vi "Auswerten.vi"(7 "Êinheiten":string[](array[string]), 8 "LIN Ausgabetabelle":refnum<vi>, 9 "Komponente:":refnum<vi>, 10 "max. Flow Weighted Mean:":refnum<vi>, 11 "Tabelle":T1[][](array[typedef])) -> (0 "Konzentration Komponente":dbl, 1 "Komponente:":T1, 2 "max. Flow Weighted Mean:":T1, 3 "Konzentration FlowWeightedMean":dbl)   [LabVIEW 2020, in "EPA 1065.lvlib" / "Interference verificaton 1065-375.lvlib"]
uses:
  Interference verificaton 1065-375.lvlib
  Visualisierungs Elemente/String - Ausgabefeld.ctl
  <vilib>/Utility/miscctls.llb/LVRowAndColumnTypeDef.ctl
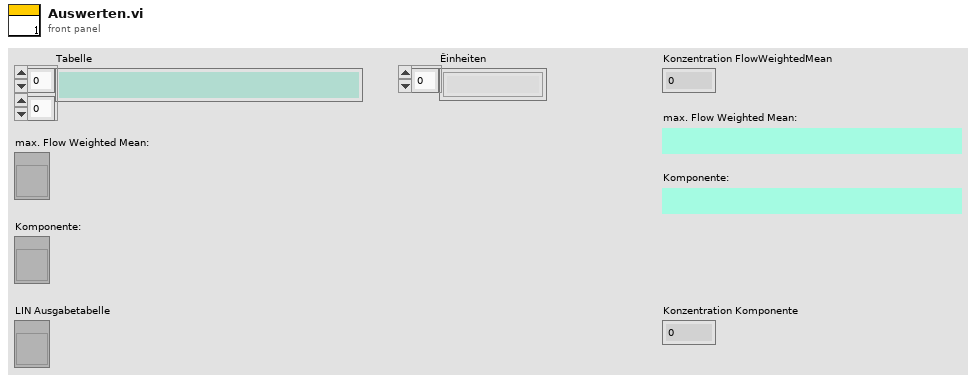
[diagram p1: front panel]
types:
  T1 = typedef "String - Ausgabefeld.ctl" = string
  T2 = typedef "LVRowAndColumnTypeDef.ctl" = cluster{"Row":i32, "Column":i32}
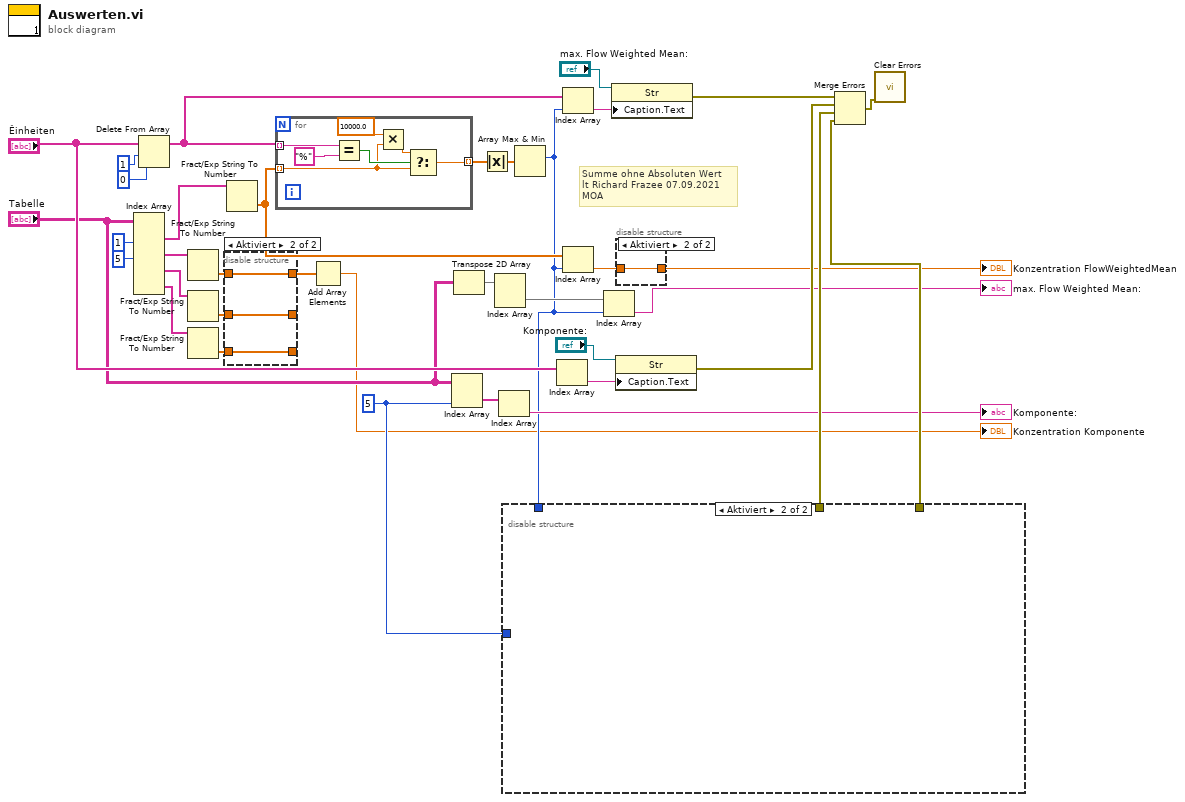
[diagram p0: block diagram]
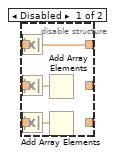
[diagram p2: hidden frame]
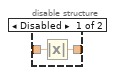
[diagram p3: hidden frame]
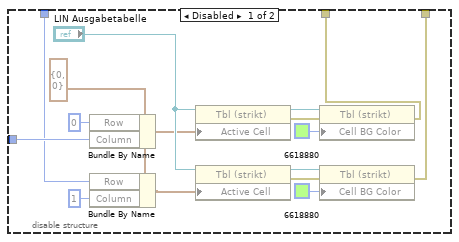
[diagram p4: hidden frame]
diagram:
  w32 = 5 ("y")
  # "Summe ohne Absoluten Wert \nlt Richard Frazee 07.09.2021\nMOA"
  n1 = Index Array(array="Tabelle", index (col) #1=1 ("Deaktivierter Index (Spalte)"), index (col) #2=5 ("Index (Spalte)")) -> (element #1=w10:T1[], element #2=w11:T1[], element #3=w14:T1[], element #4=w16:T1[])  [unwired: 6 in]
  n2 = Delete From Array(array="Êinheiten", length=1 ("Länge"), index=0 ("Index")) -> (array with subset deleted=w18:string[])  [unwired: 1 out]
  n3 = Fract/Exp String To Number(string=w11) -> (number=w12:dbl[])  [unwired: 3 in, 1 out]
  n4 = Fract/Exp String To Number(string=w14) -> (number=w13:dbl[])  [unwired: 3 in, 1 out]
  n5 = Fract/Exp String To Number(string=w16) -> (number=w15:dbl[])  [unwired: 3 in, 1 out]
  n6 = disable-structure shown="Aktiviert" {
    disable-tunnel: w15 -> [w43 w44]
    disable-tunnel: w13 -> [w42 w45]
    disable-tunnel: w12 -> [w41 w46]
    disable-tunnel: [w38 w46] -> w2
    disable-tunnel: [_ w45] -> _
    disable-tunnel: [_ w44] -> _
    frame Disabled {
      n7 = Absolute Value(x=w41) -> (abs(x)=w38:dbl[])
      n8 = Absolute Value(x=w42) -> (abs(x)=w40:dbl[])
      n9 = Absolute Value(x=w43) -> (abs(x)=w39:dbl[])
      n10 = Add Array Elements(numeric array=w40) -> ()  [unwired: 1 out]
      n11 = Add Array Elements(numeric array=w39) -> ()  [unwired: 1 out]
    }
    frame Enabled {
    }
  }
  n12 = Fract/Exp String To Number(string=w10) -> (number=w24:dbl[])  [unwired: 3 in, 1 out]
  n13 = for {
    tunnel: w18 -> [w49] mode=indexing
    tunnel: w24 -> [w48] mode=indexing
    tunnel: [w47] -> w17 mode=indexing
    n14 = Equal?(x=w49, y="%") -> (x = y?=w52:bool)
    n15 = Multiply(x=10000.0, y=w48) -> (x*y=w51:dbl)
    n16 = Select(t=w51, s=w52, f=w48) -> (s? t:f=w47:dbl)
  }
  n17 = Add Array Elements(numeric array=w2) -> (sum=→"Konzentration Komponente":dbl)
  n18 = Index Array(array="Tabelle", index (col)=w32) -> (element=w20:T1[])  [unwired: 1 in]
  n19 = Transpose 2D Array(2D array="Tabelle") -> (transposed array=w5:T1[][])
  n20 = Absolute Value(x=w17) -> (abs(x)=w4:dbl[])
  n21 = Index Array(array=w5) -> (element=w25:T1[])  [unwired: 2 in]
  n22 = Index Array(array=w20) -> (element=→"Komponente:":T1)  [unwired: 1 in]
  n23 = Array Max & Min(array=w4) -> (max index (indices)=w6:i32)  [unwired: 3 out]
  n24 = disable-structure shown="Aktiviert" {
    disable-tunnel: [w69 _] -> w37
    disable-tunnel: [w68 _] -> w36
    disable-tunnel: w32 -> [w65 _]
    disable-tunnel: w6 -> [w64 _]
    frame Disabled {
      w67 = T2 {"Row"=0, "Column"=0} ("Aktive Zelle:Aktive Zelle")
      n25 = Bundle By Name(cluster=w67, "Row"=0, "Column"=w65) -> (w58:T2)
      n26 = Bundle By Name(cluster=w67, "Row"=w64, "Column"=1) -> (w61:T2)
      n27 = property on="Eigenschaftsknoten" class="Tbl (strikt)"(reference="LIN Ausgabetabelle", "Active Cell"=w58) -> (reference out=w55:refnum<vi>, error out=w54:errorcluster)  [unwired: 1 in]
      n28 = property on="Eigenschaftsknoten" class="Tbl (strikt)"(reference="LIN Ausgabetabelle", "Active Cell"=w61) -> (reference out=w63:refnum<vi>, error out=w60:errorcluster)  [unwired: 1 in]
      n29 = property on="Eigenschaftsknoten" class="Tbl (strikt)"(reference=w55, error in=w54, "Cell BG Color"=u32 6618880) -> (error out=w68:errorcluster)  [unwired: 1 out]
      n30 = property on="Eigenschaftsknoten" class="Tbl (strikt)"(reference=w63, error in=w60, "Cell BG Color"=u32 6618880) -> (error out=w69:errorcluster)  [unwired: 1 out]
    }
    frame Enabled {
    }
  }
  n31 = Index Array(array="Êinheiten") -> (element=w23:string)  [unwired: 1 in]
  n32 = Index Array(array=w18, index=w6) -> (element=w19:string)
  n33 = Index Array(array=w24, index=w6) -> (element=w27:dbl)
  n34 = Index Array(array=w25, index=w6) -> (element=→"max. Flow Weighted Mean:":T1)
  n35 = property on="Eigenschaftsknoten" class="Str"(reference="max. Flow Weighted Mean:", "Caption.Text"=w19) -> (error out=w34:errorcluster)  [unwired: 1 in, 1 out]
  n36 = property on="Eigenschaftsknoten" class="Str"(reference="Komponente:", "Caption.Text"=w23) -> (error out=w35:errorcluster)  [unwired: 1 in, 1 out]
  n37 = disable-structure shown="Aktiviert" {
    disable-tunnel: w27 -> [w71 w72]
    disable-tunnel: [w70 w72] -> w3
    frame Disabled {
      n38 = Absolute Value(x=w71) -> (abs(x)=w70:dbl)
    }
    frame Enabled {
    }
  }
  "Konzentration FlowWeightedMean" <- w3
  n39 = Merge Errors(w34, w35, w36, w37) -> (w33:errorcluster)
  n40 = call <vilib>:"Clear Errors.vi"("error in (no error)"=w33) -> ()  [unwired: 5 in, 2 out]
